vi "DAC Save Results.vi"(8 "error in":errorcluster, 9 "Log Details?":bool, 10 "tdms file":refnum<k34>, 11 "DAC Keller Diff P 23X in":refnum<class "DAC Keller Diff P 23X.lvclass">) -> (0 "error out":errorcluster)   [LabVIEW 2019, in "DAC.lvlib" / "DAC Keller Diff P 23X.lvclass"]
uses:
  DAC Keller Diff P 23X.lvclass
  C:/Users/krio/Documents/LV_Projects/test-stand/App/DAC/DAC.lvclass
  DAC.lvclass/DAC.ctl
  DAC Keller Diff P 23X.lvclass/DAC Keller Diff P 23X.ctl
  DAC.lvclass
  <vilib>/Analysis/NI_AALBase.lvlib
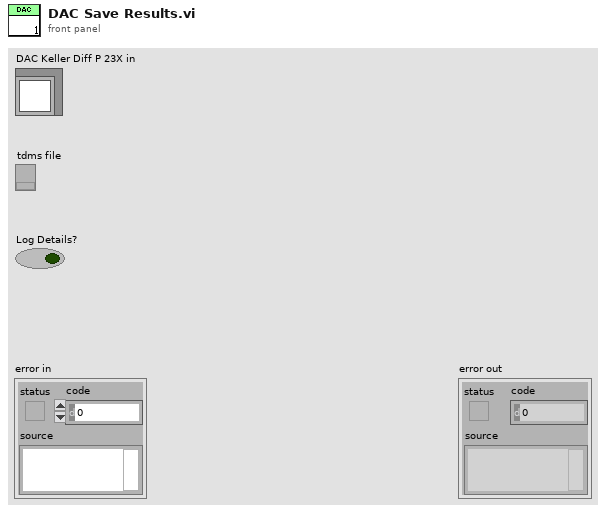
[diagram p1: front panel]
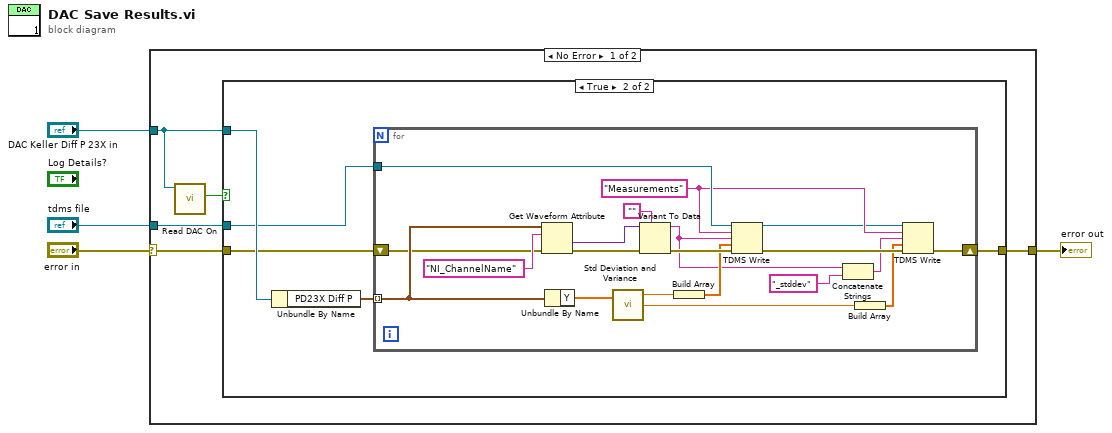
[diagram p0: block diagram]
diagram:
  n1 = case shown="No Error" "error in" {
    selector: "error in" -> [w6 w36]
    tunnel: "DAC Keller Diff P 23X in" -> [w9 _]
    tunnel: "tdms file" -> [w7 _]
    tunnel: [w5 w36] -> w1
    frame No Error {
      n2 = call "Read DAC On.vi"("DAC in"=w9) -> ("DAC On"=w8:bool)  [unwired: 8 in, 2 out]
      n3 = case shown="True" w8 {
        tunnel: w9 -> [_ w15]
        tunnel: w7 -> [_ w14]
        tunnel: w6 -> [w10 w13]
        tunnel: [w10 w12] -> w5
        frame False {
        }
        frame True {
          n4 = Unbundle By Name(w15) -> ("PD23X Diff P"=w11:waveform(dbl)[])
          n5 = for {
            tunnel: w14 -> [w35]
            tunnel: w11 -> [w31] mode=indexing
            shift-right: [w23] -> w12
            shift-left: w13 -> [w30]
            w22 = "Measurements" ("group name in (Untitled)")
            n6 = Get Waveform Attribute(4:w30, 6:"NI_ChannelName" ("name"), 7:w31) -> (0:w29:errorcluster, 1:w33:variant)  [unwired: 1 in, 2 out]
            n7 = Unbundle By Name(w31) -> ("Y"=w27:dbl[])
            n8 = call <vilib>:"Std Deviation and Variance.vi"("X"=w27) -> ("mean"=w26:dbl, "standard deviation"=w20:dbl)  [unwired: 1 in, 1 out]
            n9 = Variant To Data(error in=w29, type="", Variant=w33) -> (data=w18:string, error out=w28:errorcluster)
            n10 = Build Array(w26) -> (w25:dbl[])
            n11 = TDMS Write(0:w35, 5:w22, 7:w18, 9:w25, 11:w28) -> (4:w21:refnum<k34>, 15:w24:errorcluster)  [unwired: 1 in, 2 out]
            n12 = Concatenate Strings(w18, "_stddev" ("string")) -> (w16:string)
            n13 = Build Array(w20) -> (w19:dbl[])
            n14 = TDMS Write(0:w21, 5:w22, 7:w16, 9:w19, 11:w24) -> (15:w23:errorcluster)  [unwired: 1 in, 3 out]
          }
        }
      }
    }
    frame Error {
    }
  }
  "error out" <- w1
